vi "Define Default Prefix.vi"(8 "error in":errorcluster, 11 "PWM input channel in":refnum<class "PWM Input Channel.lvclass">) -> (0 "error out":errorcluster, 3 "PWM input channel out":refnum<class "PWM Input Channel.lvclass">)   [LabVIEW 2017, in "Scan Engine Scripting.lvlib" / "PWM Input Channel.lvclass"]
uses:
  PWM Input Channel.lvclass
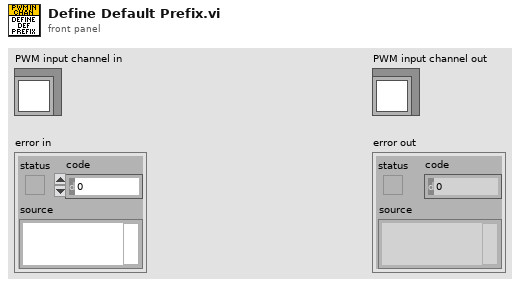
[diagram p1: front panel]
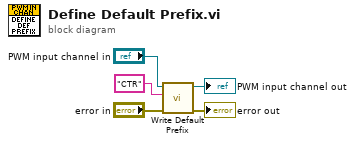
[diagram p0: block diagram]
diagram:
  n1 = call-dynamic "Write Default Prefix.vi"("error in"="error in", "default prefix"="CTR", "channel in"="PWM input channel in") -> ("error out"=→"error out":errorcluster, "channel out"=→"PWM input channel out":refnum<class "PWM Input Channel.lvclass">)  [unwired: 7 in]
